vi "mon exit logic.vi"(0 "temp":T1 {"utility"."therm volt" format="%_6g"; "utility"."heat volt in" format="%_6g"; "utility"."heat volt out" format="%_6g"; "utility"."power out" format="%_6g"; "utility"."H Vmax" format="%_6g"; "T exec"."man power" format="%_6g"; "T exec"."exec setpoint" format="%_6g"; "T params"."Settle Time" step=1.0; "T params"."Settle Bandwidth" step=0.01; "T params"."Derivative Tme" step=0.01; "T params"."Integral Time" step=1.0; "T params"."Control Bandwidth" step=0.1; "T params"."Setpoint" step=0.1; "T status"."Setpoint" format="%_6g"; "T status"."Power" format="%_6g"; "T status"."Temp" format="%_6g"}, 11 "error in (no error)":errorcluster, 12 "sec":bool, 13 "early exit":bool) -> (4 "temp out":T1 {"utility"."therm volt" format="%_6g"; "utility"."heat volt in" format="%_6g"; "utility"."heat volt out" format="%_6g"; "utility"."power out" format="%_6g"; "utility"."H Vmax" format="%_6g"; "T exec"."man power" format="%_6g"; "T exec"."exec setpoint" format="%_6g"; "T params"."Settle Time" step=1.0; "T params"."Settle Bandwidth" step=0.01; "T params"."Derivative Tme" step=0.01; "T params"."Integral Time" step=1.0; "T params"."Control Bandwidth" step=0.1; "T params"."Setpoint" step=0.1; "T status"."Setpoint" format="%_6g"; "T status"."Power" format="%_6g"; "T status"."Temp" format="%_6g"}, 8 "T mode":T3, 14 "exit loop":bool, 15 "error out":errorcluster)   [LabVIEW 2019]
doc: "This is a Bug C(T) subVI.\n\nIt handles the exit logic for the monitor loop.\n\nPaul K Dixon\nP3600\nCSUSB Physics"
uses:
  typedefs/temp cont cluster.ctl
  typedefs/temp exec cluster.ctl
  typedefs/temp mode enum.ctl
  typedefs/temp indicator.ctl
  typedefs/temp control status.ctl
  typedefs/PID control parameters.ctl
  typedefs/temp cont utility.ctl
  globals/Bug globals.vi
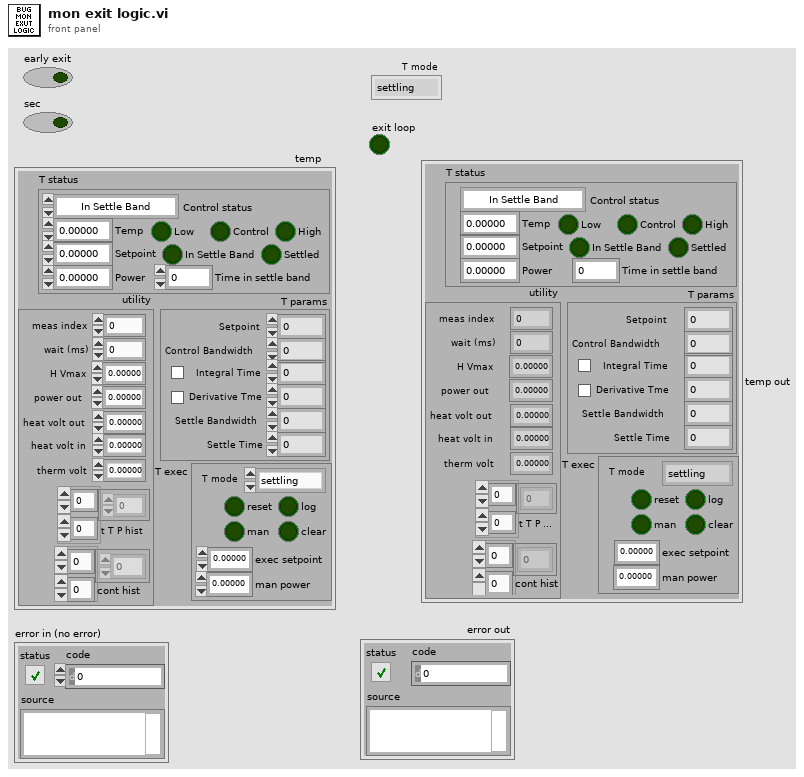
[diagram p1: front panel]
types:
  T1 = typedef "temp cont cluster.ctl" = cluster{"T exec":T2, "T status":T4, "T params":T6, "utility":T7}
  T2 = typedef "temp exec cluster.ctl" = cluster{"T mode":T3, "exec setpoint":dbl, "reset":bool, "man power":dbl, "man":bool, "log":bool, "clear":bool}
  T3 = typedef "temp mode enum.ctl" = enum16{"settling", "measuring", "holding", "Exit"}
  T4 = typedef "temp indicator.ctl" = cluster{"Control status":T5, "Temp":dbl, "Power":dbl, "Time in settle band":dbl, "Settled":bool, "Low":bool, "High":bool, "Setpoint":dbl, "Control":bool, "In Settle Band":bool}
  T5 = typedef "temp control status.ctl" = enum16{"In Settle Band", "In Control Band", "Below Control Band", "Above Control Band"}
  T6 = typedef "PID control parameters.ctl" = cluster{"Setpoint":dbl, "Control Bandwidth":dbl, "Integral Time":dbl, "Int\nON":bool, "Derivative Tme":dbl, "Der\nON":bool, "Settle Bandwidth":dbl, "Settle Time":dbl}
  T7 = typedef "temp cont utility.ctl" = cluster{"meas index":i32, "wait (ms)":i32, "H Vmax":dbl, "power out":dbl, "heat volt out":dbl, "heat volt in":dbl, "therm volt":dbl, "t T P hist":dbl[][], "cont hist":dbl[][]}
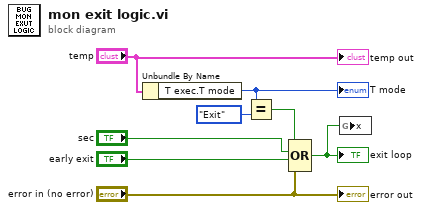
[diagram p0: block diagram]
diagram:
  n1 = Unbundle By Name("temp") -> ("T exec.T mode"=w7:T3)
  "T mode" <- w7
  n2 = Equal?(x=w7, y=temp_mode_enum."Exit" ("exec.T mode")) -> (x = y?=w3:bool)
  n3 = Compound Arithmetic op=OR(w3, "sec", "early exit", "error in (no error)") -> (w1:bool)
  "exit loop" <- w1
  n4 = global write "Bug globals.vi" "x"(w1) -> ()
  "error out" <- "error in (no error)"
  "temp out" <- "temp"
